vi "Formula Node.vi"(1 "c":dbl, 2 "b":dbl, 3 "a":dbl, 4 "x":dbl) -> (0 "f":dbl)   [LabVIEW 2025]
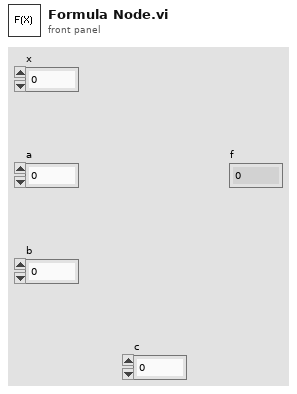
[diagram p1: front panel]
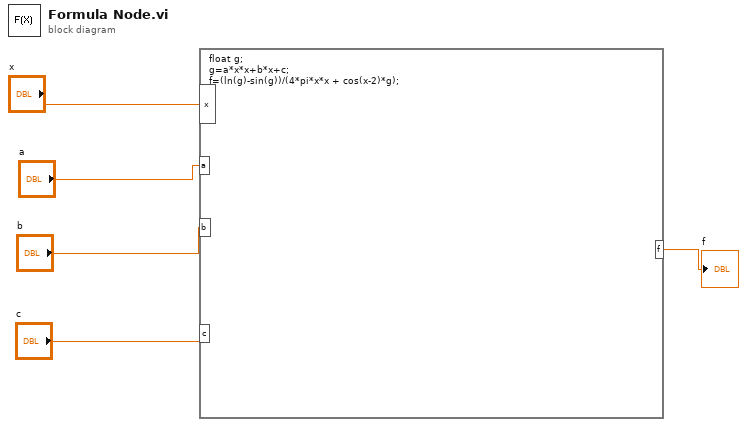
[diagram p0: block diagram]
diagram:
  n1 = formula code="float g;\ng=a*x*x+b*x+c;\nf=(ln(g)-sin(g))/(4*pi*x*x + cos(x-2)*g);"("x"="x", "a"="a", "b"="b", "c"="c") -> ("f"=→"f":dbl)
